vi "Gif._Example.vi"() -> ()   [LabVIEW 2019]
doc: "The Example vi calls the Main vi. It will play the animation until the user stops it."
panel:
  in  "image index":i32=-1
  out "element":picture
  out "error out":errorcluster
  in  "stop":bool
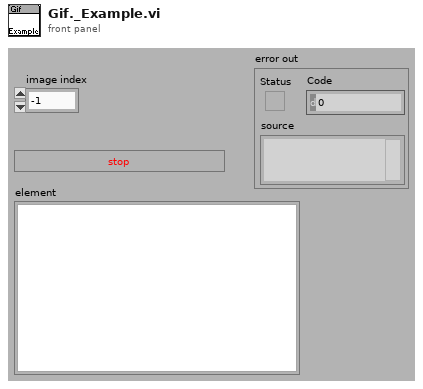
[diagram p1: front panel]
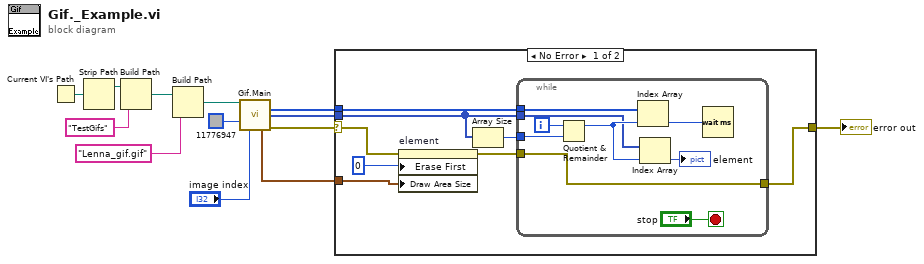
[diagram p0: block diagram]
diagram:
  n1 = Current VI's Path() -> (path=w8:path)
  n2 = Strip Path(path=w8) -> (stripped path=w7:path)  [unwired: 1 out]
  n3 = Build Path(base path=w7, name or relative path="TestGifs" ("Name oder relativer Pfad")) -> (appended path=w3:path)
  n4 = Build Path(base path=w3, name or relative path="Lenna_gif.gif" ("Name oder relativer Pfad")) -> (appended path=w5:path)
  n5 = call "Gif.Main.vi"("file path"=w5, "bgcolor"=u32 11776947, "image index"="image index") -> ("time"=w13:u32[], "images out"=w2:picture[], "image size"=w12:cluster{"Width":u32, "Height":u32}, "error out"=w11:errorcluster)  [unwired: 1 in, 8 out]
  n6 = case shown="No Error" w11 {
    selector: w11 -> [w16 w31]
    tunnel: w13 -> [w19 _]
    tunnel: w12 -> [w14 _]
    tunnel: [w20 w31] -> w10
    tunnel: w2 -> [w18 _]
    frame No Error {
      n7 = property on="element" class="Pict"(error in=w16, "Erase First"=u8 0 ("Zuerst löschen"), "Draw Area Size"=w14) -> (error out=w15:errorcluster)  [unwired: 1 in, 1 out]
      n8 = Array Size(array=w18) -> (size(s)=w21:i32)
      n9 = while {
        tunnel: w19 -> [w24]
        tunnel: w15 -> [w26]
        tunnel: w21 -> [w28]
        tunnel: [w26] -> w20
        tunnel: w18 -> [w23]
        i -> [w29]
        stop <- "stop" stop-if-true
        n10 = Quotient & Remainder(x=w29, y=w28) -> (x-y*floor(x/y)=w27:i32)  [unwired: 1 out]
        n11 = Index Array(array=w24, index=w27) -> (element=w25:u32)
        n12 = Index Array(array=w23, index=w27) -> (element=→"element":picture)
        n13 = Wait (ms)(milliseconds to wait=w25) -> ()  [unwired: 1 out]
      }
    }
    frame Error {
    }
  }
  "error out" <- w10
